vi "Puzzle 18-2.vi"() -> ()   [LabVIEW 2022 SP3]
panel:
  in  "delimited string":string="L 4 (#906400)\nD 13 (#01d963)\nL 3 (#79a0e0)\nU 10 (#98a913)\nL 2 (#19c840)\nU 3 (#47db23)\nL 4 (#a84580)\nU 4 (#5bac33)\nL 6 (#58c070)\nU 6 (#089513)\nL 9 (#1dfa20)\nU 2 (#3c5e23)\nL 4 (#621d52)\nU 6 (#bf9c73)\nL 9 (#50eb22)\nU 2 (#286a93)\nL 3 (#72d9e2)\nU 5 (#806033)\nL 3 (#832ce0)\nU 5 (#8e26b3)\nL 2 (#30d5f2)\nU 13 (#97a923)\nL 3 (#5256f2)\nU 4 (#154f63)\nL 11 (#42ed72)\nU 6 (#368651)\nL 7 (#21fb22)\nU 6 (#5ff031)\nL 7 (#89bf92)\nU 7 (#6a91c1)\nL 7 (#89bf90)\nU 6 (#a12501)\nL 5 (#21fb20)\nU 6 (#195221)\nL 6 (#514db2)\nU 6 (#a750f1)\nL 8 (#3af182)\nU 6 (#a750f3)\nL 2 (#4dbe42)\nU 4 (#4cd933)\nL 6 (#ad8800)\nU 4 (#390b13)\nL 5 (#6d56f2)\nU 3 (#279653)\nL 3 (#94fa52)\nU 5 (#31efe3)\nL 4 (#45ce10)\nU 10 (#4d3ab3)\nL 7 (#7286e0)\nU 9 (#280e23)\nL 4 (#49fc50)\nU 6 (#6debc3)\nL 5 (#a72fe0)\nU 3 (#36c9e3)\nL 5 (#46f620)\nU 4 (#448f13)\nL 8 (#2ca942)\nU 6 (#555aa3)\nL 5 (#399532)\nU 5 (#483083)\nL 10 (#7cec72)\nU 6 (#5ebe53)\nL 3 (#686db2)\nU 5 (#0040d3)\nL 8 (#0e2ba2)\nU 7 (#8803d3)\nL 9 (#00bbc2)\nU 6 (#8e6a03)\nL 7 (#1120f2)\nU 3 (#522df3)\nR 6 (#512a82)\nU 9 (#3f0631)\nR 7 (#019a30)\nU 3 (#b94321)\nR 7 (#019a32)\nU 3 (#6d6821)\nR 3 (#a469d2)\nU 5 (#4d6dc1)\nR 7 (#824c22)\nU 4 (#1f1d73)\nR 3 (#2b5402)\nU 3 (#9b1593)\nR 10 (#28b092)\nU 3 (#114f43)\nR 8 (#595422)\nU 7 (#506211)\nR 8 (#014122)\nU 2 (#aa8581)\nR 2 (#7b5922)\nU 9 (#0efde1)\nR 3 (#39c632)\nU 5 (#6e3a61)\nL 4 (#7d8012)\nU 4 (#159383)\nR 4 (#15bc72)\nU 6 (#6cb663)\nR 7 (#444262)\nU 6 (#52c351)\nR 4 (#9800c2)\nU 3 (#52c353)\nL 4 (#012572)\nU 7 (#1811b3)\nL 6 (#5e8a32)\nU 4 (#6f1fd3)\nL 3 (#3df5c0)\nU 11 (#6b3d23)\nL 3 (#3295d0)\nU 6 (#639293)\nL 6 (#6208c0)\nU 3 (#5a3581)\nL 4 (#212042)\nU 4 (#27a8c1)\nR 3 (#212040)\nU 2 (#4cf171)\nR 9 (#0d87d0)\nU 4 (#437a43)\nR 7 (#719310)\nU 5 (#2b2a33)\nR 3 (#1bd8d2)\nU 7 (#61c453)\nR 2 (#1f4e80)\nU 4 (#08b443)\nL 9 (#9726c0)\nU 6 (#2a7373)\nL 6 (#57ba80)\nU 10 (#653173)\nL 6 (#13e8e0)\nU 4 (#985921)\nL 7 (#86f4d0)\nU 5 (#85d8a3)\nL 4 (#5bf682)\nD 9 (#27b353)\nL 4 (#09c1c0)\nU 9 (#0ecf63)\nL 6 (#a15350)\nU 6 (#0ecf61)\nR 7 (#2d3af0)\nU 3 (#2673a3)\nR 2 (#b2e500)\nU 6 (#620613)\nR 7 (#0f6bd0)\nD 3 (#1c7543)\nR 2 (#0a10c0)\nD 6 (#59ae93)\nR 3 (#9506a0)\nD 5 (#37f853)\nR 7 (#5e29f0)\nU 5 (#597243)\nR 5 (#a47a52)\nU 3 (#140b03)\nR 2 (#a47a50)\nU 6 (#67b023)\nR 10 (#0068b0)\nD 6 (#0a4aa3)\nR 9 (#3ab5c0)\nD 8 (#79a163)\nR 5 (#64c650)\nD 6 (#44cad3)\nR 6 (#51e700)\nD 3 (#56c053)\nL 9 (#09ce80)\nD 2 (#1ea873)\nL 2 (#73dff2)\nD 9 (#a29b21)\nR 8 (#2d4522)\nD 5 (#a29b23)\nL 6 (#4d00f2)\nD 5 (#42ec53)\nL 4 (#bc5c20)\nD 8 (#21f071)\nL 4 (#8a6f10)\nD 5 (#5591f1)\nR 3 (#0a3b82)\nD 12 (#2e3e01)\nR 4 (#9aa5c0)\nD 8 (#8ea681)\nR 7 (#9aa5c2)\nD 5 (#602721)\nL 8 (#0a3b80)\nD 4 (#0f16d1)\nR 2 (#a2deb0)\nD 11 (#2d2ee1)\nR 6 (#21a420)\nU 6 (#5da871)\nR 6 (#4f3d80)\nU 7 (#c0da91)\nR 3 (#4f3d82)\nU 6 (#011b91)\nR 3 (#41ff40)\nU 2 (#4c1ec1)\nR 7 (#af4f10)\nU 2 (#06dcd1)\nR 6 (#0ebc70)\nU 4 (#0a9051)\nR 7 (#653602)\nU 3 (#6e9211)\nR 4 (#606072)\nU 5 (#39fc01)\nL 10 (#c59670)\nU 7 (#3ffb51)\nR 9 (#063452)\nU 3 (#61fc51)\nR 4 (#6b83b2)\nU 5 (#0b4801)\nL 9 (#48e9b2)\nU 3 (#a22491)\nL 4 (#457ea2)\nU 4 (#018051)\nL 8 (#24bc42)\nD 7 (#80bb31)\nR 5 (#4c5392)\nD 11 (#120631)\nL 5 (#9f7850)\nD 4 (#653a83)\nL 9 (#c3ae60)\nU 2 (#653a81)\nL 3 (#0e0970)\nU 4 (#67c3e1)\nR 7 (#7395d0)\nU 8 (#4c1161)\nL 7 (#6cd100)\nU 4 (#0d6c03)\nR 7 (#388930)\nU 8 (#220913)\nR 4 (#415690)\nU 7 (#5ea4a3)\nR 8 (#5d8712)\nU 8 (#9b9393)\nR 5 (#5d8710)\nU 3 (#002983)\nL 4 (#7dc760)\nU 8 (#1e52f3)\nL 9 (#025a00)\nD 8 (#1c1253)\nL 3 (#b789a0)\nU 3 (#1c1251)\nL 4 (#1b78d0)\nU 8 (#0bb5a3)\nR 6 (#4d6930)\nU 11 (#367da3)\nR 2 (#c8f352)\nU 3 (#44cc63)\nR 8 (#c8f350)\nD 3 (#5ac933)\nL 5 (#207e60)\nD 5 (#85afe3)\nR 5 (#01d742)\nD 6 (#902b33)\nR 4 (#1e5032)\nU 5 (#854b81)\nR 4 (#6df0c2)\nU 2 (#5e92e1)\nR 7 (#64a4f2)\nD 5 (#078fa1)\nR 3 (#730962)\nD 5 (#078fa3)\nR 2 (#146262)\nD 5 (#2b2f93)\nR 11 (#1e8282)\nD 2 (#b8aed3)\nR 11 (#05b2d2)\nD 2 (#902b31)\nR 6 (#2500c2)\nD 6 (#0af8a3)\nR 4 (#778c32)\nD 5 (#8ffe83)\nR 6 (#4b59f0)\nU 5 (#1bc403)\nR 5 (#680210)\nD 8 (#355103)\nR 4 (#6f0f40)\nD 3 (#4f8da3)\nR 5 (#0193c0)\nD 4 (#1236b3)\nR 3 (#24a310)\nD 7 (#7d9383)\nR 3 (#a7aa90)\nD 5 (#065c93)\nR 3 (#59e070)\nD 4 (#99e113)\nR 6 (#28f8d0)\nU 4 (#4c8283)\nR 3 (#200c10)\nU 5 (#2f3d13)\nR 6 (#a0a790)\nD 5 (#744603)\nR 4 (#30a200)\nD 8 (#82bdd3)\nR 5 (#7b0d50)\nU 5 (#15a7c1)\nR 3 (#7410f2)\nU 7 (#5308c1)\nR 4 (#54de30)\nD 9 (#74b971)\nR 4 (#54de32)\nD 3 (#355941)\nR 3 (#7410f0)\nD 6 (#1a9561)\nR 4 (#5666b0)\nD 3 (#7c2b23)\nR 6 (#ac6ab0)\nD 10 (#3c6181)\nR 4 (#479482)\nU 9 (#4b3c11)\nR 7 (#5be122)\nU 5 (#44f8a1)\nL 6 (#9474a2)\nU 3 (#7c8f11)\nL 7 (#579ed0)\nU 3 (#70fb11)\nR 13 (#98b6f0)\nU 4 (#16d6c1)\nL 7 (#479480)\nU 8 (#27cf11)\nR 6 (#6a5de0)\nD 2 (#a6cf63)\nR 9 (#1c2240)\nD 3 (#535b63)\nR 4 (#ba5b40)\nD 2 (#3a70a3)\nR 5 (#1c07e2)\nD 7 (#328f03)\nL 9 (#90b982)\nD 7 (#4e78e3)\nR 3 (#29bc22)\nD 3 (#4322e3)\nL 2 (#409ea0)\nD 3 (#19c8f3)\nL 7 (#7b3e20)\nD 4 (#925493)\nL 5 (#2c7b40)\nD 5 (#ac1d81)\nL 7 (#081b90)\nD 2 (#27a361)\nL 4 (#1bf3d0)\nD 5 (#295af3)\nL 12 (#957dd0)\nD 5 (#00e5a3)\nR 4 (#432960)\nD 2 (#a44e43)\nR 8 (#0e2e60)\nD 9 (#0711a1)\nR 6 (#9e8d70)\nD 6 (#68fac1)\nR 3 (#9e8d72)\nU 4 (#5e8271)\nR 7 (#1c7e80)\nD 4 (#27a363)\nR 4 (#5a19c0)\nD 7 (#069561)\nL 6 (#334990)\nD 3 (#069563)\nL 5 (#67dd80)\nD 9 (#7c2b21)\nL 2 (#3a0ed0)\nD 2 (#ad5d33)\nL 7 (#1e84e0)\nD 7 (#2edbc1)\nL 6 (#74b590)\nU 7 (#0e1491)\nL 6 (#504080)\nD 5 (#0e1493)\nL 4 (#a9f120)\nU 8 (#2edbc3)\nL 8 (#251b40)\nD 8 (#ad5d31)\nL 3 (#5ed770)\nD 5 (#3ae671)\nL 7 (#061552)\nU 4 (#009981)\nL 5 (#0ca222)\nU 9 (#23b031)\nR 7 (#496292)\nU 5 (#16ec01)\nR 7 (#8ee312)\nU 4 (#67a321)\nR 4 (#24a272)\nD 4 (#16c0f1)\nR 4 (#1cc622)\nU 7 (#7fcff1)\nL 3 (#a7fd32)\nU 5 (#789b91)\nL 2 (#3358a0)\nU 5 (#5322b1)\nL 7 (#922a90)\nD 10 (#835913)\nL 3 (#603690)\nU 4 (#835911)\nL 7 (#3d4130)\nU 3 (#078c81)\nL 4 (#0ef3f0)\nD 2 (#adc831)\nL 3 (#6273f0)\nD 11 (#39f881)\nL 5 (#17c6a0)\nD 4 (#b7d2a1)\nL 6 (#17c6a2)\nD 3 (#4a4ff1)\nR 10 (#7d5902)\nD 6 (#8aa763)\nL 10 (#15f8e2)\nD 6 (#0d8e93)\nL 6 (#8b98e2)\nD 8 (#428061)\nL 5 (#2c9832)\nD 5 (#579bb1)\nR 5 (#453452)\nD 4 (#5acad3)\nR 5 (#3477b2)\nU 3 (#3f5143)\nR 7 (#5fb842)\nU 3 (#6b4553)\nR 9 (#3dcbb2)\nD 7 (#247d53)\nR 4 (#166552)\nU 4 (#5e9e53)\nR 3 (#765a32)\nU 5 (#920223)\nR 5 (#5c4fb2)\nD 5 (#2609c3)\nR 7 (#15bf50)\nD 4 (#201523)\nR 7 (#bcea90)\nD 8 (#6309f3)\nR 5 (#3e6cb2)\nD 12 (#726c23)\nR 5 (#536492)\nD 5 (#1509d3)\nR 5 (#808d92)\nD 4 (#7fe721)\nR 2 (#06eca0)\nD 9 (#5caa21)\nR 4 (#3105e0)\nU 13 (#939171)\nR 4 (#3105e2)\nU 5 (#244431)\nR 3 (#06eca2)\nD 4 (#991be1)\nR 9 (#8f3eb2)\nD 8 (#3f4591)\nR 6 (#4a8e22)\nU 4 (#a8cd41)\nR 2 (#430fb2)\nU 7 (#33a231)\nR 7 (#602992)\nU 7 (#68bf81)\nL 10 (#7ee6c2)\nU 4 (#7cd521)\nR 10 (#a42412)\nU 5 (#1ee571)\nR 2 (#039072)\nU 12 (#516221)\nR 4 (#60e3c2)\nD 5 (#bb8851)\nR 7 (#60e3c0)\nD 3 (#81ab81)\nR 5 (#8e80c2)\nD 4 (#18e071)\nR 5 (#943bc0)\nU 9 (#6a5b41)\nR 2 (#76ef70)\nU 3 (#70c4c1)\nR 5 (#7d7fb0)\nU 5 (#a0cb51)\nR 4 (#1ed780)\nD 8 (#4f9261)\nR 2 (#9bbcf0)\nD 5 (#138771)\nR 3 (#823170)\nD 4 (#673221)\nR 11 (#72fd30)\nD 6 (#3354e3)\nR 8 (#347150)\nD 8 (#3354e1)\nR 8 (#49ea60)\nD 4 (#5baca1)\nR 3 (#20a250)\nD 3 (#55d6f1)\nL 11 (#269a70)\nD 6 (#514711)\nR 7 (#641a30)\nD 7 (#a25ba1)\nR 5 (#641a32)\nD 4 (#211b51)\nL 8 (#8dbb20)\nD 3 (#0efcf1)\nL 4 (#02fe80)\nD 4 (#4476b3)\nR 2 (#296da0)\nD 4 (#774ca3)\nR 9 (#ad0dc0)\nD 5 (#052723)\nR 8 (#196740)\nD 3 (#62d083)\nR 6 (#4dc8c0)\nD 4 (#9d8ee1)\nR 3 (#4684a2)\nD 11 (#749641)\nL 3 (#778490)\nD 8 (#170271)\nL 6 (#6b1c40)\nD 5 (#4bbdc1)\nL 8 (#4d5bf0)\nD 6 (#71d7b1)\nR 4 (#363800)\nD 3 (#3540b1)\nR 4 (#6eed72)\nD 9 (#6b9861)\nR 2 (#2f1cc2)\nD 2 (#0c9551)\nR 5 (#a39e42)\nU 5 (#0c9553)\nL 4 (#248c52)\nU 6 (#5cbe01)\nR 4 (#4684a0)\nU 3 (#49e411)\nR 5 (#147d02)\nD 8 (#22e8e1)\nR 7 (#47c702)\nD 5 (#6a7721)\nR 3 (#6b0a62)\nD 4 (#8d6003)\nR 6 (#143e92)\nD 10 (#3686f3)\nR 7 (#594052)\nU 6 (#7dcf03)\nR 5 (#19e8d2)\nU 7 (#2ac123)\nR 4 (#7c8732)\nU 4 (#59a753)\nR 5 (#3e4872)\nU 9 (#6e0623)\nR 3 (#767cf2)\nD 4 (#476623)\nR 2 (#00e3b2)\nD 5 (#799291)\nR 8 (#4fb4f2)\nD 2 (#7e14a1)\nR 4 (#44e8b2)\nD 3 (#6ff981)\nL 10 (#03c9e0)\nD 6 (#4c0a11)\nL 4 (#03c9e2)\nD 6 (#3a7fe1)\nR 5 (#73a822)\nD 7 (#782481)\nR 6 (#1fced2)\nD 8 (#5164e1)\nL 7 (#18fa22)\nD 7 (#00ac93)\nL 5 (#0af5c0)\nD 3 (#200ee3)\nL 3 (#244172)\nD 6 (#a5dc13)\nR 10 (#244170)\nD 4 (#129e13)\nL 8 (#0af5c2)\nD 4 (#266773)\nL 2 (#64a1a2)\nD 4 (#1bcf13)\nL 7 (#5ade72)\nU 3 (#74f681)\nL 4 (#1c7b92)\nU 6 (#95f3d1)\nR 4 (#1c7b90)\nU 5 (#1081c1)\nL 2 (#600742)\nU 4 (#a4da11)\nL 8 (#56b352)\nU 6 (#5dd011)\nL 3 (#41b240)\nD 6 (#142841)\nL 6 (#298cc0)\nD 6 (#1dee71)\nR 8 (#2dfda0)\nD 4 (#863f61)\nR 2 (#7b0ee0)\nD 11 (#2a7fd1)\nR 4 (#70c8d2)\nD 7 (#7ed441)\nR 9 (#97faa2)\nD 4 (#7ed443)\nR 3 (#0b8812)\nD 5 (#380fd1)\nL 12 (#2bbaf2)\nD 3 (#3797b1)\nL 8 (#101d22)\nU 3 (#bbd851)\nL 9 (#101d20)\nU 6 (#3f9731)\nL 4 (#10fda0)\nD 8 (#2bd171)\nL 3 (#15fa90)\nD 4 (#c30771)\nL 4 (#15fa92)\nU 8 (#971561)\nL 3 (#10fda2)\nU 4 (#09b3c1)\nL 3 (#771bd2)\nU 9 (#a74c31)\nL 7 (#480c62)\nU 7 (#31c003)\nL 7 (#32b6b2)\nU 7 (#4db183)\nL 5 (#315702)\nD 7 (#01ac13)\nL 5 (#6d3812)\nU 7 (#3c9253)\nL 8 (#47c7a0)\nU 3 (#396c93)\nL 10 (#47c7a2)\nU 3 (#589283)\nL 3 (#25e122)\nD 6 (#476671)\nL 5 (#2520d2)\nU 9 (#1658c1)\nL 4 (#7905c2)\nU 5 (#5ec5d1)\nL 7 (#638e42)\nU 8 (#9329f1)\nL 2 (#367a42)\nU 7 (#448cd3)\nL 6 (#47c8e2)\nU 7 (#53c891)\nR 8 (#3e9d00)\nU 7 (#757191)\nR 5 (#3e9d02)\nD 3 (#05c551)\nR 2 (#386ca2)\nD 10 (#7a87b3)\nR 6 (#1c60d2)\nD 6 (#5477c3)\nR 5 (#5db422)\nU 3 (#7cc273)\nR 4 (#67ea02)\nU 4 (#a53143)\nR 7 (#204b80)\nU 4 (#4a7073)\nL 3 (#447c70)\nU 3 (#72cad3)\nL 8 (#7a4fa0)\nU 5 (#72cad1)\nR 6 (#3bcc70)\nU 4 (#625903)\nL 3 (#2cc5d0)\nU 10 (#acc971)\nL 3 (#1a8aa0)\nU 3 (#2a9173)\nL 3 (#a6cb80)\nD 9 (#53f763)\nL 3 (#a6cb82)\nD 4 (#5fc703)\nL 3 (#4338e0)\nU 7 (#9e8b23)\nL 7 (#4338e2)\nU 5 (#8699f3)\nL 10 (#159e12)\nU 5 (#1b3de3)\nL 8 (#1e5802)\nU 6 (#06c193)\nL 9 (#691102)\nU 5 (#9e6e43)\nL 4 (#32bb52)\nU 7 (#8ce3a3)\nL 6 (#0c5e72)\nU 2 (#11c163)\nL 3 (#20d7b2)\nD 9 (#3aa213)\nL 5 (#a25cd2)\nD 4 (#397da3)\nL 4 (#2b3e82)\nD 3 (#2f1353)\nL 8 (#503842)\nD 5 (#6d25b1)\nL 11 (#a55782)\nD 5 (#6d25b3)\nR 11 (#008022)\nD 6 (#2e3033)\nL 3 (#2574b2)\nD 6 (#9d58f3)\nL 6 (#841200)\nD 4 (#296673)\nL 2 (#c2b110)\nD 5 (#5e07e3)\nL 8 (#5b1262)\nD 3 (#0c1b43)\nL 8 (#27cf52)\nD 4 (#0c1b41)\nR 7 (#4b46b2)\nD 5 (#4848b3)\nR 6 (#2d7c52)\nD 3 (#3818e3)\nR 4 (#3c5792)\nU 8 (#06a691)\nR 7 (#18dc52)\nD 8 (#c55b81)\nL 3 (#2a8582)\nD 5 (#2d58a3)\nL 6 (#46f8a2)\nD 9 (#9ea973)\nL 4 (#375002)\nD 3 (#56daf3)\nL 4 (#7f15d2)\nU 7 (#177923)\nL 3 (#627e82)\nU 5 (#713b83)\nL 3 (#416152)\nD 9 (#51edb3)\nL 2 (#a3dfd0)\nD 2 (#7b8423)\nL 7 (#631ce2)\nD 9 (#a54f53)\nR 4 (#2be612)\nD 3 (#282a71)\nR 5 (#861152)\nD 6 (#476751)\nR 4 (#4683f2)\nD 2 (#7d2b31)\nR 8 (#1a7222)\nD 3 (#51f383)\nL 10 (#32f982)\nD 3 (#6f40f3)\nL 11 (#32f980)\nD 4 (#2b8883)\nL 9 (#54c132)\nD 8 (#239bb3)\nL 6 (#0ff5c2)\nU 4 (#09a3f3)"
  out "integral(ydx)":dbl
  out "appended array":cluster{"row":i32, "col":i32}[](array[cluster])
  out "Array":string[](array[string])
  out "Array 2":u64[](array[numeric])
  out "Array":string[](array[string])
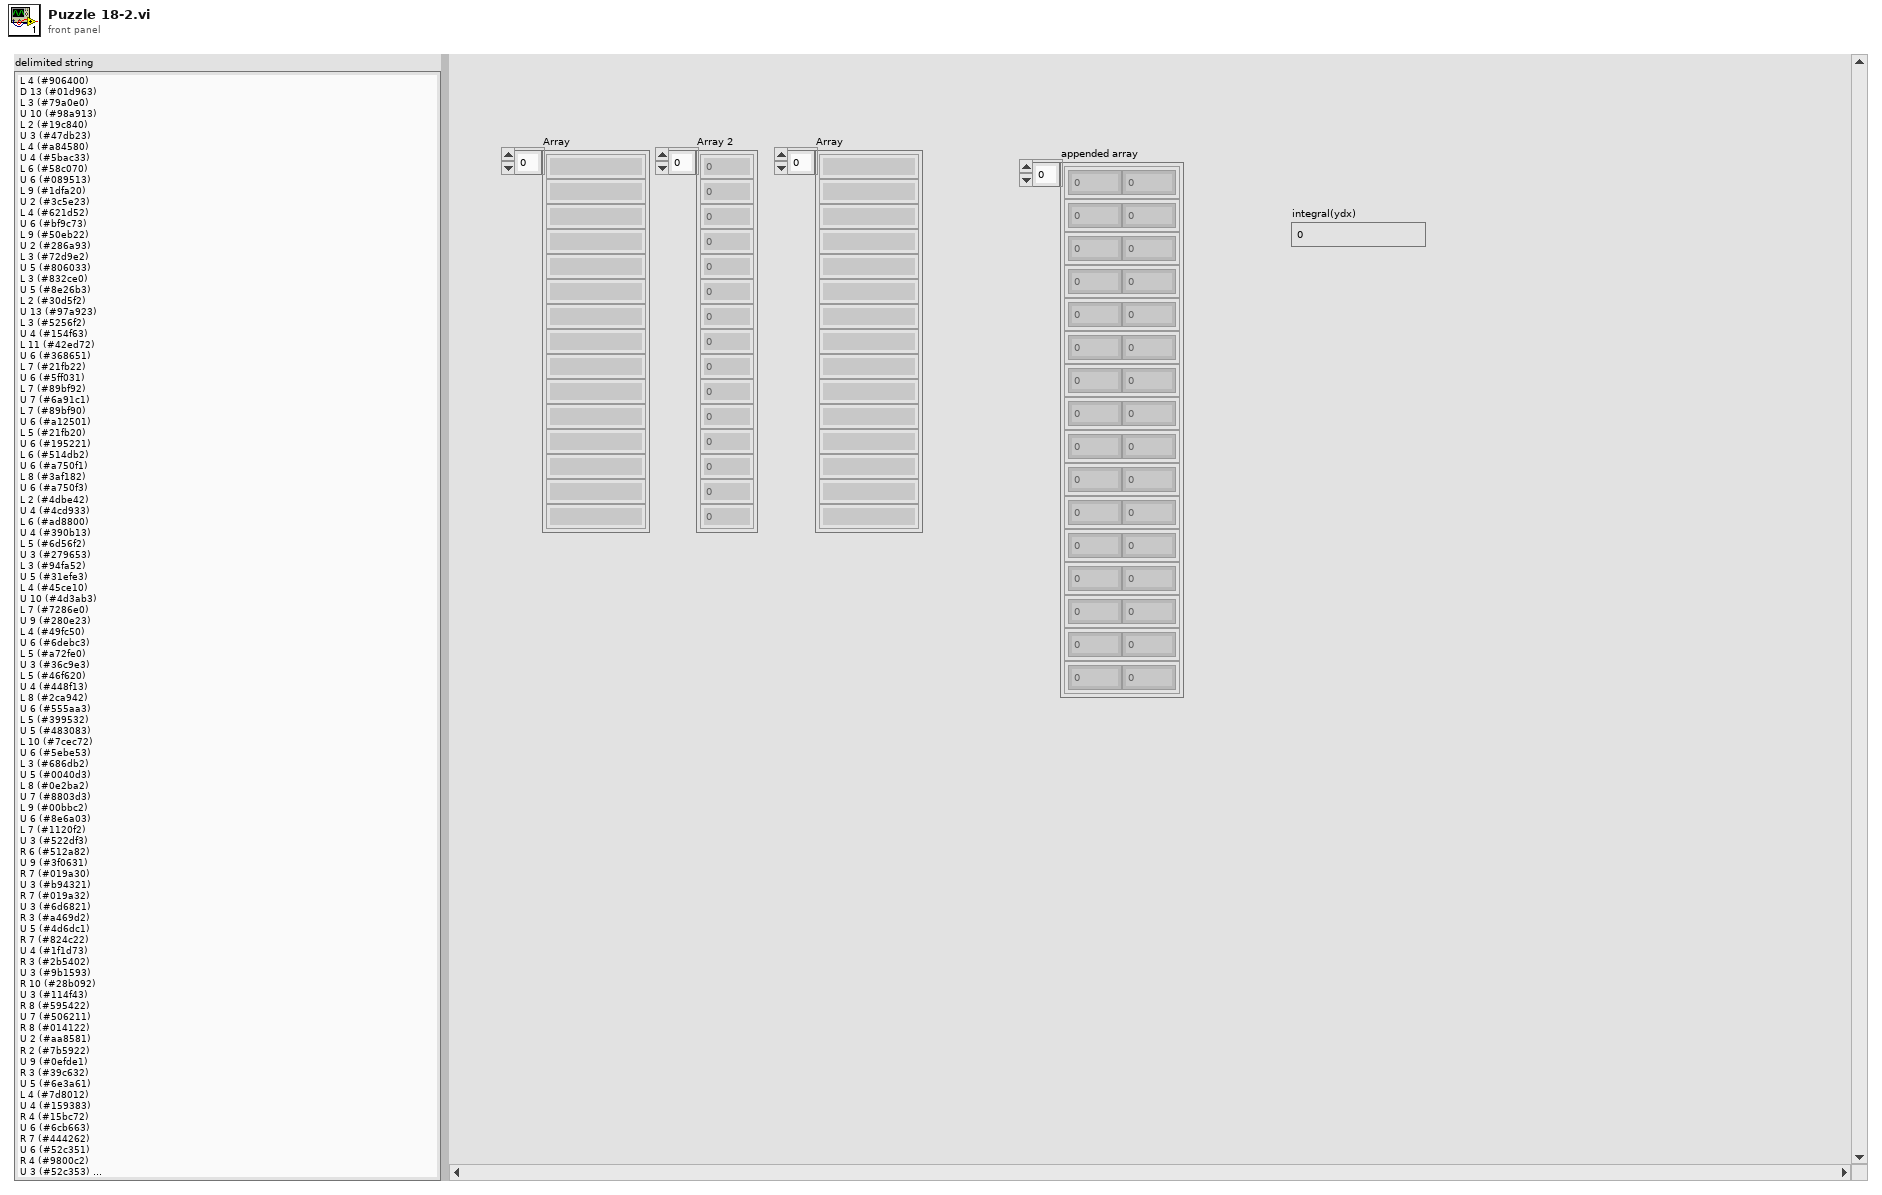
[diagram p1: front panel]
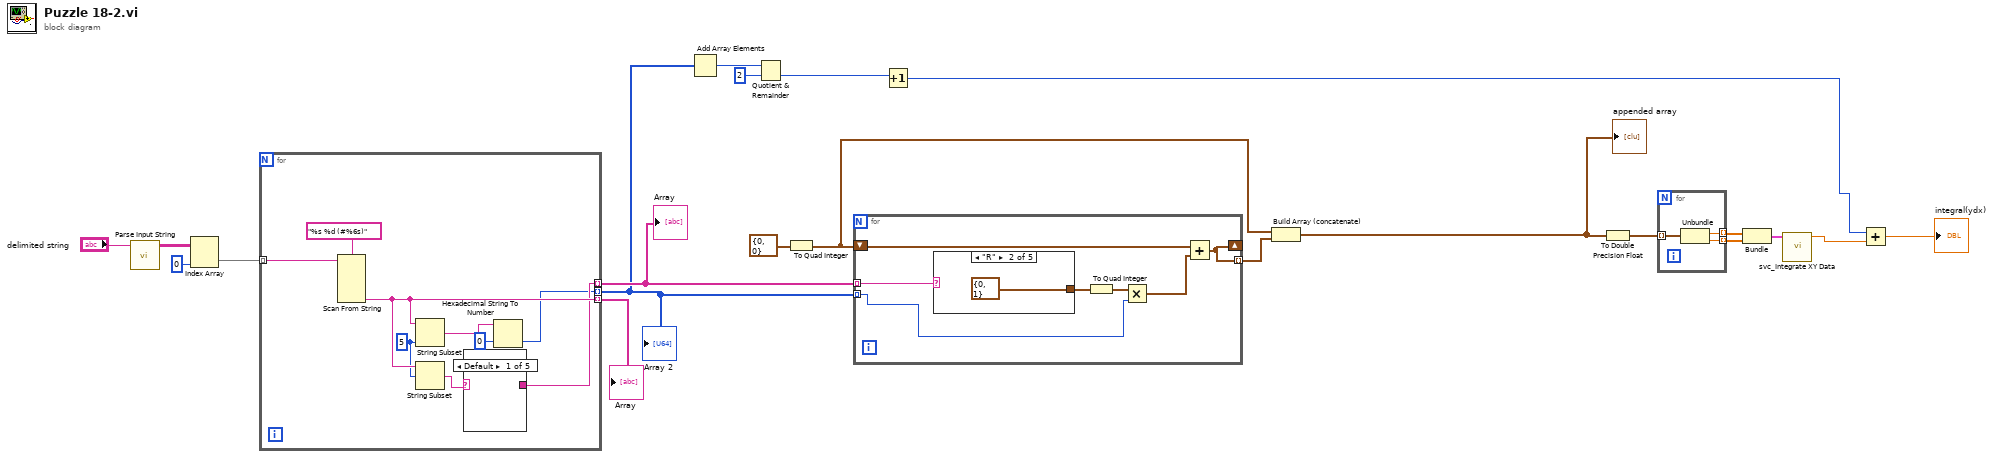
[diagram p0: block diagram]
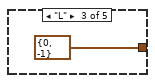
[diagram p3: hidden frame]
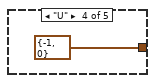
[diagram p4: hidden frame]
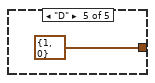
[diagram p5: hidden frame]
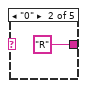
[diagram p6: hidden frame]
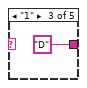
[diagram p7: hidden frame]
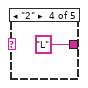
[diagram p8: hidden frame]
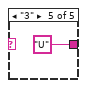
[diagram p9: hidden frame]
diagram:
  n1 = call "Parse Input String.vi"("delimited string"="delimited string") -> ("parsed string"=w20:string[][])  [unwired: 10 in]
  n2 = Index Array(array=w20, index (col)=0 ("disabled index (col)")) -> (element=w18:string[])  [unwired: 1 in]
  n3 = for {
    tunnel: w18 -> [w30] mode=indexing
    tunnel: [w24] -> w10 mode=indexing
    tunnel: [w23] -> w2 mode=indexing
    tunnel: [w27] -> w9 mode=indexing
    w26 = 5 ("length (rest)")
    n4 = Scan From String(format string="%s %d (#%6s)", input string=w30) -> (output 3=w27:string)  [unwired: 7 in, 3 out]
    n5 = String Subset(string=w27, length (rest)=w26) -> (substring=w28:string)  [unwired: 1 in]
    n6 = String Subset(string=w27, offset (0)=w26) -> (substring=w25:string)  [unwired: 1 in]
    n7 = case shown="Default" w25 {
      tunnel: [_ "R" ("format string") "D" ("format string") "L" ("format string") "U" ("format string")] -> w24
      frame Default {
      }
      frame "0" {
      }
      frame "1" {
      }
      frame "2" {
      }
      frame "3" {
      }
    }
    n8 = Hexadecimal String To Number(string=w28, default (0uL)=i64 0 ("default (0 U32)")) -> (number=w23:i64)  [unwired: 1 in, 1 out]
  }
  "Array" <- w10
  "Array 2" <- w2
  "Array" <- w9
  n9 = Add Array Elements(numeric array=w2) -> (sum=w8:i64)
  n10 = Quotient & Remainder(x=w8, y=u64 2) -> (floor(x/y)=w6:u64)  [unwired: 1 out]
  n11 = To Quad Integer(1:cluster{"row":i64, "col":i64} {"row"=0, "col"=0}) -> (0:w1:cluster{"row":i64, "col":i64})
  n12 = for {
    shift-right: [w38] -> _
    shift-left: w1 -> [w39]
    tunnel: w10 -> [w41] mode=indexing
    tunnel: w2 -> [w36] mode=indexing
    tunnel: [w38] -> w17 mode=indexing
    n13 = case shown="\"R\"" w41 {
      tunnel: [_ cluster{"row":i32, "col":i32} {"row"=0, "col"=1} cluster{"row":i32, "col":i32} {"row"=0, "col"=-1} cluster{"row":i32, "col":i32} {"row"=-1, "col"=0} cluster{"row":i32, "col":i32} {"row"=1, "col"=0}] -> w40
      frame Default {
      }
      frame "R" {
      }
      frame "L" {
      }
      frame "U" {
      }
      frame "D" {
      }
    }
    n14 = To Quad Integer(1:w40) -> (0:w35:cluster{"row":i64, "col":i64})
    n15 = Multiply(x=w35, y=w36) -> (x*y=w37:cluster{"row":i64, "col":i64})
    n16 = Add(x=w39, y=w37) -> (x+y=w38:cluster{"row":i64, "col":i64})
  }
  n17 = Increment(x=w6) -> (x+1=w4:u64)
  n18 = Build Array (concatenate)(w1, w17) -> (w16:cluster{"row":i64, "col":i64}[])
  "appended array" <- w16
  n19 = To Double Precision Float(number=w16) -> (double precision float=w15:cluster{"row":dbl, "col":dbl}[])
  n20 = for {
    tunnel: w15 -> [w48] mode=indexing
    tunnel: [w47] -> w14 mode=indexing
    tunnel: [w46] -> w13 mode=indexing
    n21 = Unbundle(w48) -> ("row"=w47:dbl, "col"=w46:dbl)
  }
  n22 = Bundle(w14, w13) -> (w12:cluster{dbl[], dbl[]})  [unwired: 1 in]
  n23 = call <vilib>:"svc_Integrate XY Data.vi"("XY"=w12) -> ("integral(ydx)"=w5:dbl)  [unwired: 10 in]
  n24 = Add(x=w4, y=w5) -> (x+y=→"integral(ydx)":dbl)
